vi "GUI - Stop Test (SubVI).vi"(7 "References":T1) -> ()   [LabVIEW 2010]
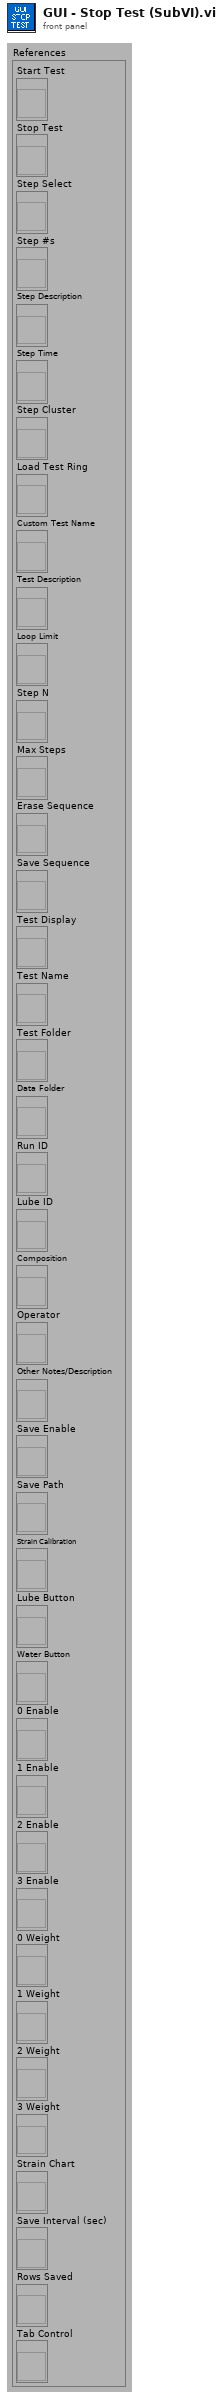
[diagram p1: front panel]
types:
  T1 = cluster{"Start Test":refnum<vi>, "Stop Test":refnum<vi>, "Step Select":refnum<vi>, "Step #s":refnum<vi>, "Step Description":refnum<vi>, "Step Time":refnum<vi>, "Step Cluster":refnum<vi>, "Load Test Ring":refnum<vi>, "Custom Test Name":refnum<vi>, "Test Description":refnum<vi>, "Loop Limit":refnum<vi>, "Step N":refnum<vi>, "Max Steps":refnum<vi>, "Erase Sequence":refnum<vi>, "Save Sequence":refnum<vi>, "Test Display":refnum<vi>, "Test Name":refnum<vi>, "Test Folder":refnum<vi>, "Data Folder":refnum<vi>, "Run ID":refnum<vi>, "Lube ID":refnum<vi>, "Composition":refnum<vi>, "Operator":refnum<vi>, "Other Notes/Description":refnum<vi>, "Save Enable":refnum<vi>, "Save Path":refnum<vi>, "Strain Calibration":refnum<vi>, "Lube Button":refnum<vi>, "Water Button":refnum<vi>, "0 Enable":refnum<vi>, "1 Enable":refnum<vi>, "2 Enable":refnum<vi>, "3 Enable":refnum<vi>, "0 Weight":refnum<vi>, "1 Weight":refnum<vi>, "2 Weight":refnum<vi>, "3 Weight":refnum<vi>, "Strain Chart":refnum<vi>, "Save Interval (sec)":refnum<vi>, "Rows Saved":refnum<vi>, "Tab Control":refnum<vi>}
  T2 = enum8{"Enabled", "Disabled", "Disabled and Grayed Out"}
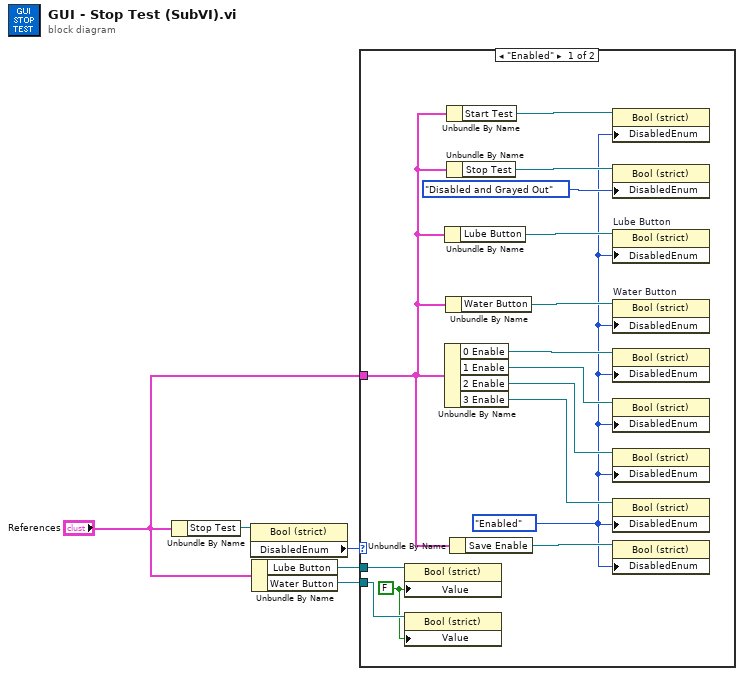
[diagram p0: block diagram]
diagram:
  n1 = Unbundle By Name("References") -> ("Stop Test"=w5:refnum<vi>)
  n2 = property class="Bool (strict)"(reference=w5) -> ("DisabledEnum"=w2:T2)  [unwired: 1 in, 2 out]
  n3 = Unbundle By Name("References") -> ("Lube Button"=w3:refnum<vi>, "Water Button"=w4:refnum<vi>)
  n4 = case shown="\"Enabled\"" w2 {
    tunnel: w3 -> [w20 _]
    tunnel: w4 -> [w19 _]
    tunnel: "References" -> [w8 _]
    frame "Enabled" {
      w6 = T2."Enabled" ("Disabled")
      w18 = FALSE
      n5 = property class="Bool (strict)"(reference=w20, "Value"=w18) -> ()  [unwired: 1 in, 2 out]
      n6 = property class="Bool (strict)"(reference=w19, "Value"=w18) -> ()  [unwired: 1 in, 2 out]
      n7 = Unbundle By Name(w8) -> ("Lube Button"=w13:refnum<vi>)
      n8 = Unbundle By Name(w8) -> ("0 Enable"=w17:refnum<vi>, "1 Enable"=w16:refnum<vi>, "2 Enable"=w15:refnum<vi>, "3 Enable"=w14:refnum<vi>)
      n9 = Unbundle By Name(w8) -> ("Water Button"=w12:refnum<vi>)
      n10 = Unbundle By Name(w8) -> ("Start Test"=w9:refnum<vi>)
      n11 = Unbundle By Name(w8) -> ("Stop Test"=w10:refnum<vi>)
      n12 = Unbundle By Name(w8) -> ("Save Enable"=w7:refnum<vi>)
      n13 = property class="Bool (strict)"(reference=w9, "DisabledEnum"=w6) -> ()  [unwired: 1 in, 2 out]
      n14 = property class="Bool (strict)"(reference=w10, "DisabledEnum"=T2."Disabled and Grayed Out") -> ()  [unwired: 1 in, 2 out]
      n15 = property on="Lube Button" class="Bool (strict)"(reference=w13, "DisabledEnum"=w6) -> ()  [unwired: 1 in, 2 out]
      n16 = property on="Water Button" class="Bool (strict)"(reference=w12, "DisabledEnum"=w6) -> ()  [unwired: 1 in, 2 out]
      n17 = property class="Bool (strict)"(reference=w17, "DisabledEnum"=w6) -> ()  [unwired: 1 in, 2 out]
      n18 = property class="Bool (strict)"(reference=w16, "DisabledEnum"=w6) -> ()  [unwired: 1 in, 2 out]
      n19 = property class="Bool (strict)"(reference=w15, "DisabledEnum"=w6) -> ()  [unwired: 1 in, 2 out]
      n20 = property class="Bool (strict)"(reference=w14, "DisabledEnum"=w6) -> ()  [unwired: 1 in, 2 out]
      n21 = property class="Bool (strict)"(reference=w7, "DisabledEnum"=w6) -> ()  [unwired: 1 in, 2 out]
    }
    frame "Disabled", Default {
    }
  }
